vi "Test Example Password 1.vi"() -> ()   [LabVIEW 2014]
panel:
  out "isPasswordLocked?":bool
  in  "Error In":errorcluster
  in  "vi path":path=path "C:/Users/ljagos/Documents/LabVIEW/LabVIEW-Universal-Transcriptor/Test/Examples For Parsing/Example Variant Info.vi"
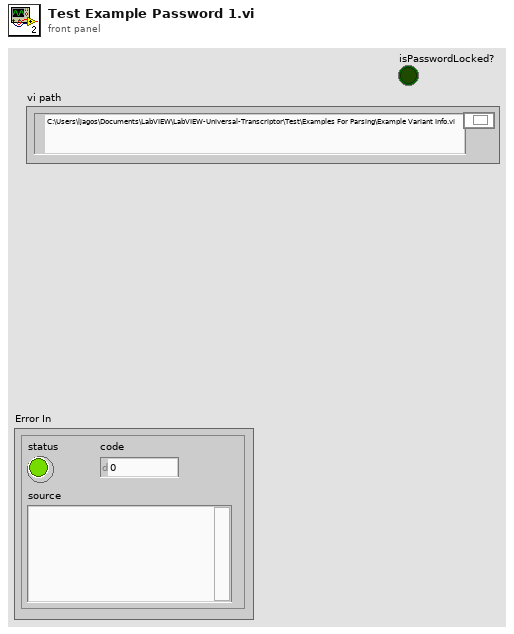
[diagram p1: front panel]
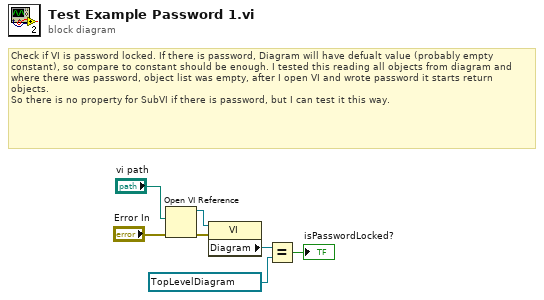
[diagram p0: block diagram]
diagram:
  # "Check if VI is password locked. If there is password, Diagram will have defualt value (probably empty constant), so compare to constant should be enough. I tested this reading all objects from diagram and where there was password, object list was empty, after I open VI and wrote password it starts return objects.\nSo there is no property for SubVI if there is password, but I can test it this way."
  n1 = Open VI Reference(vi path="vi path", error in (no error)="Error In") -> (vi reference=w4:refnum<vi>, error out=w5:errorcluster)  [unwired: 4 in]
  n2 = property class="VI"(reference=w4, error in=w5) -> ("Diagram"=w2:refnum<vi>)  [unwired: 2 out]
  n3 = Equal?(x=w2, y=refnum<vi> refnum ("Block Diagram")) -> (x = y?=→"isPasswordLocked?":bool)
